vi "read_dust_control_settings.vi"(7 "Settings to be loaded":i32, 8 "error in (no error)":errorcluster, 9 "Cluster":T1, 10 "Lower Timestamp Range":timestamp, 11 "Upper Timestamp Range":timestamp) -> (0 "error out":errorcluster, 1 "Array":cluster{"String":string, "Value":dbl}[](array[cluster]), 3 "Dust Source Array":T2[](array[typedef]) {"Needle Voltage" min=0.0 max=10.0 step=0.01 format="%.2g"; "Y Voltage" min=0.0 max=9.0 step=0.01 format="%.2g"; "X Voltage" min=0.0 max=9.0 step=0.01 format="%.2g"; "Einzel Voltage" min=0.0 max=10.0 step=0.01 format="%.2g"; "Desired Amplitude (V)" min=0.0 max=10.0 step=0.01 format="%5.2f"; "Width (ms) : 0.1" min=0.05 max=5.0 step=0.01 format="%6.2f"; "Frequency" min=1.0 max=100.0 step=0.01 format="%.1f"})   [LabVIEW 2013]
uses:
  Controls/dust_soruce_control.ctl
  <vilib>/addons/database/Auxilliary.llb/DB Tools Cursor Type.ctl
  <vilib>/addons/database/Connection.llb/Conn Execute.vi
  <vilib>/addons/database/Recordset.llb/Rec Fetch Recordset Data (R).vi
  <vilib>/addons/database/Recordset.llb/Rec Destroy - Connection.vi
  <vilib>/addons/database/_DB Variant To Data/Database Variant To Data.xnode
  <vilib>/addons/database/NI_Database_API.lvlib
panel:
  out "Settings ID 2":dbl(ring) caption="Settings ID" items=["Auto", "Auto", "Auto", "Auto", "Auto", "Auto", "Auto", "Auto", "Auto", "Auto", "Auto", "Auto", "Auto", "Auto", "Auto", "Auto", "Auto", "Auto", "Auto", "Auto", "Auto test", "Auto", "Automatic Update at  10/19/2012 4:35:52 PM", "Automatic Update at  10/19/2012 4:37:24 PM", "Automatic Update at  10/19/2012 4:37:56 PM", "Automatic Update at  10/19/2012 4:39:59 PM", "Automatic Update at  10/19/2012 4:40:46 PM", "Automatic Update at  10/19/2012 4:43:56 PM", "Automatic Update at  10/19/2012 5:03:34 PM", "Awesome settings that work", "Awesome settings that work", "Automatic Update at  10/19/2012 5:32:08 PM", "Automatic Update at  10/19/2012 5:34:15 PM", "Automatic Update at  10/19/2012 5:39:51 PM", "Working settings", "Working settings", "Working settings", "Working settings", "Working settings", "Automatic Update at  10/22/2012 1:18:52 PM", "Automatic Update at  10/22/2012 1:22:32 PM", "", "Test", "Test", "Automatic Update at  10/22/2012 1:29:56 PM", "Test", "Test 1", "Test 1", "Anna's Settings", "Automatic Update at  10/22/2012 3:57:19 PM", "test of width", "Automatic Update at  10/22/2012 4:02:00 PM", "Automatic Update at  10/22/2012 4:10:30 PM", "Automatic Update at  10/22/2012 4:15:00 PM", "Automatic Update at  10/22/2012 4:38:33 PM", "Automatic Update at  10/22/2012 4:44:48 PM", "Automatic Update at  10/22/2012 4:46:11 PM", "Automatic Update at  10/22/2012 4:51:36 PM", "Automatic Update at  10/22/2012 4:54:36 PM", "Automatic Update at  10/22/2012 4:59:09 PM", "Automatic Update at  10/22/2012 5:01:02 PM", "Automatic Update at  10/22/2012 5:06:29 PM", "Automatic Update at  10/22/2012 5:13:46 PM", "Automatic Update at  10/22/2012 5:18:54 PM", "Automatic Update at  10/22/2012 5:27:58 PM", "Automatic Update at  10/22/2012 5:37:45 PM", "Automatic Update at  10/22/2012 5:39:44 PM", "Automatic Update at  10/22/2012 5:41:21 PM", "Automatic Update at  10/22/2012 5:41:55 PM", "Automatic Update at  10/22/2012 5:43:41 PM", "Automatic Update at  10/22/2012 5:45:31 PM", "Anna's Settings (Updated with working Giraffes)", "Anna's Settings (Updated with working Giraffes)", "Automatic Update at  10/23/2012 1:01:38 PM", "test", "test", "test 1", "test 1", "Automatic Update at  10/23/2012 1:44:56 PM", "Automatic Update at  10/23/2012 1:52:29 PM", "Automatic Update at  10/23/2012 1:59:24 PM", "test 3", "test 4", "Automatic Update at  10/23/2012 2:20:20 PM", "Automatic Update at  10/23/2012 5:53:49 PM", "Anna's Settings", "Anna's Settings1", "test mctesty", "test mctesty", "Automatic Update at  10/24/2012 3:47:44 PM", "Test\"", "Test\"", "this is a \"test\" setting", "Automatic Update at  10/24/2012 4:13:56 PM"]
  out "SQL Query Sintax":string
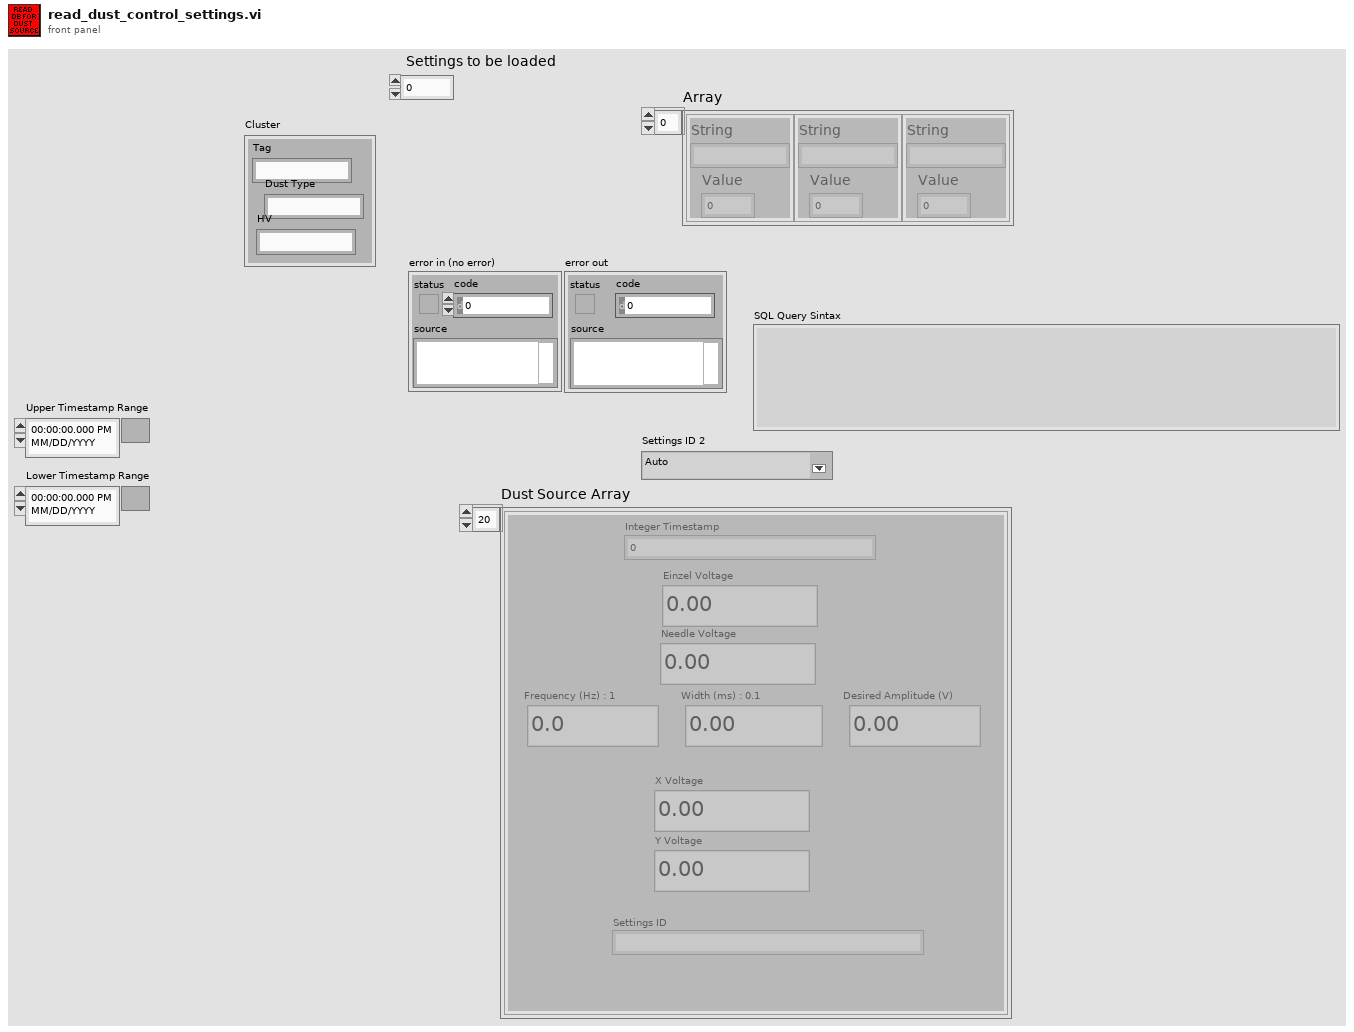
[diagram p1: front panel]
types:
  T1 = cluster{"Tag":string, "Dust Type":string, "HV":string}
  T2 = typedef "dust_soruce_control.ctl" = cluster{"Integer Timestamp":u64, "Einzel Voltage":dbl, "Needle Voltage":dbl, "Frequency":dbl, "Width (ms) : 0.1 ":dbl, "Desired Amplitude (V)":dbl, "X Voltage":dbl, "Y Voltage":dbl, "Settings ID":string, "ID#":i32}
  T3 = typedef "NI_Database_API.lvlib/DB Tools Cursor Type.ctl" = enum16{"forward-only", "keyset", "dynamic", "static"}
  T4 = typedef "NI_Database_API.lvlib/Conn ObjectReference.ctl" = refnum<k1>
  T5 = typedef "NI_Database_API.lvlib/Rec ObjectReference.ctl" = refnum<k1>
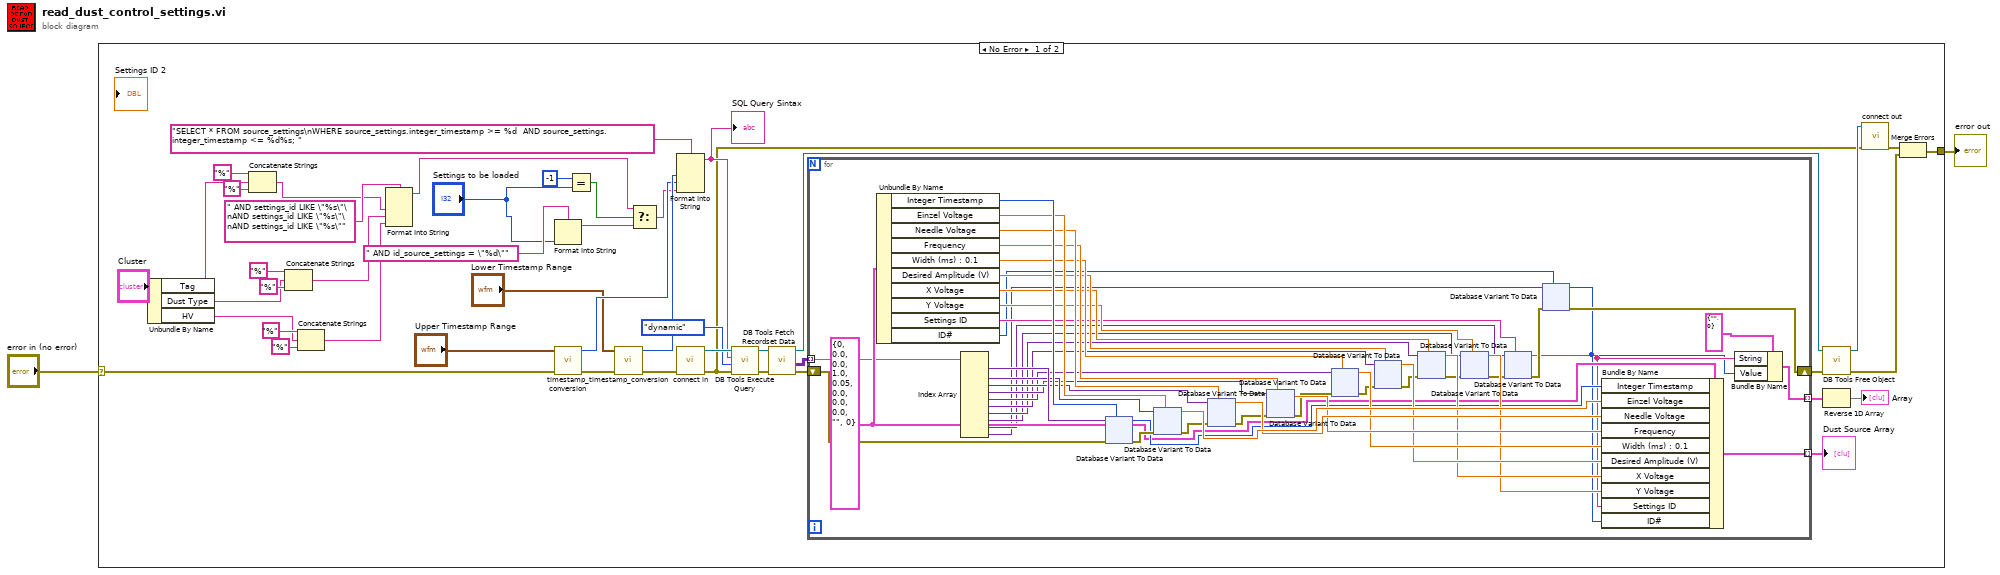
[diagram p0: block diagram]
diagram:
  n1 = case shown="No Error" "error in (no error)" {
    selector: "error in (no error)" -> [w39 w415]
    tunnel: [w22 w415] -> w1
    frame No Error {
      n2 = Unbundle By Name("Cluster") -> ("Tag"=w11:string, "Dust Type"=w6:string, "HV"=w7:string)
      n3 = Concatenate Strings("%" ("string"), w11, "%" ("string")) -> (w14:string)
      n4 = Concatenate Strings("%" ("string"), w6, "%" ("string")) -> (w4:string)
      n5 = Concatenate Strings("%" ("string"), w7, "%" ("string")) -> (w3:string)
      n6 = Format Into String(format string=" AND settings_id LIKE \"%s\"\nAND settings_id LIKE \"%s\"\nAND settings_id LIKE \"%s\"" ("string"), w14, w4, w3) -> (resulting string=w13:string)  [unwired: 2 in, 1 out]
      n7 = Format Into String(format string=" AND id_source_settings = \"%d\"" ("string"), "Settings to be loaded") -> (resulting string=w35:string)  [unwired: 2 in, 1 out]
      n8 = call "timestamp_conversion.vi"("error in (no error)"=w39, "Time Stamp"="Upper Timestamp Range") -> ("error out"=w40:errorcluster, "Integer Time"=w33:i64)  [unwired: 7 in]
      n9 = Equal?(x=-1, y="Settings to be loaded") -> (x = y?=w41:bool)
      n10 = call "timestamp_conversion.vi"("error in (no error)"=w40, "Time Stamp"="Lower Timestamp Range") -> ("error out"=w37:errorcluster, "Integer Time"=w34:i64)  [unwired: 7 in]
      n11 = Select(t=w13, s=w41, f=w35) -> (s? t:f=w27:string)
      n12 = Format Into String(format string="SELECT * FROM source_settings\nWHERE source_settings.integer_timestamp >= %d  AND source_settings.integer_timestamp <= %d%s; " ("string"), w34, w33, w27) -> (resulting string=w31:string)  [unwired: 2 in, 1 out]
      "SQL Query Sintax" <- w31
      n13 = call "connect in.vi"("error in (no error)"=w37) -> ("error out"=w20:errorcluster, "Database Connection"=w43:T4)  [unwired: 6 in, 1 out]
      n14 = call-poly <vilib>:"DB Tools Execute Query.vi"("error in (no error)"=w20, "cursor type"=DB_Tools_Cursor_Type."dynamic", "SQL query"=w31, "connection reference"=w43) -> ("error out"=w47:errorcluster, "recordset reference"=w48:T5)  [unwired: 4 in]
      n15 = call-poly <vilib>:"DB Tools Fetch Recordset Data.vi"("error in (no error)"=w47, "recordset reference"=w48) -> ("error out"=w45:errorcluster, "recordset data"=w38:variant[][], "recordset reference out"=w46:T5)  [unwired: 3 in]
      n16 = for {
        tunnel: w38 -> [w75] mode=indexing
        shift-right: [w55] -> w44
        shift-left: w45 -> [w94]
        tunnel: [w78] -> w26 mode=indexing
        tunnel: [w51] -> w25 mode=indexing
        w76 = T2 {"Integer Timestamp"=0, "Einzel Voltage"=0.0, "Needle Voltage"=0.0, "Frequency"=1.0, "Width (ms) : 0.1 "=0.05, "Desired Amplitude (V)"=0.0, "X Voltage"=0.0, "Y Voltage"=0.0, "Settings ID"="", "ID#"=0} ("Dust Source Controls")
        n17 = Unbundle By Name(w76) -> ("Integer Timestamp"=w74:u64, "Einzel Voltage"=w72:dbl, "Needle Voltage"=w70:dbl, "Frequency"=w68:dbl, "Width (ms) : 0.1"=w66:dbl, "Desired Amplitude (V)"=w63:dbl, "X Voltage"=w61:dbl, "Y Voltage"=w60:dbl, "Settings ID"=w58:string, "ID#"=w53:i32)
        n18 = Index Array(array=w75) -> (element #1=w73:variant, element #2=w71:variant, element #3=w69:variant, element #4=w67:variant, element #5=w65:variant, element #6=w64:variant, element #7=w62:variant, element #8=w59:variant, element #9=w57:variant, element #10=w54:variant)  [unwired: 10 in]
        n19 = xnode "Database Variant To Data"("database variant"=w73, "error in"=w94, "type"=w74) -> ("data"=w77:u64, "error out"=w92:errorcluster)
        n20 = xnode "Database Variant To Data"("database variant"=w71, "error in"=w92, "type"=w72) -> ("data"=w93:dbl, "error out"=w90:errorcluster)
        n21 = xnode "Database Variant To Data"("database variant"=w69, "error in"=w90, "type"=w70) -> ("data"=w91:dbl, "error out"=w88:errorcluster)
        n22 = xnode "Database Variant To Data"("database variant"=w67, "error in"=w88, "type"=w68) -> ("data"=w89:dbl, "error out"=w86:errorcluster)
        n23 = xnode "Database Variant To Data"("database variant"=w65, "error in"=w86, "type"=w66) -> ("data"=w87:dbl, "error out"=w85:errorcluster)
        n24 = xnode "Database Variant To Data"("database variant"=w64, "error in"=w85, "type"=w63) -> ("data"=w84:dbl, "error out"=w82:errorcluster)
        n25 = xnode "Database Variant To Data"("database variant"=w62, "error in"=w82, "type"=w61) -> ("data"=w83:dbl, "error out"=w80:errorcluster)
        n26 = xnode "Database Variant To Data"("database variant"=w59, "error in"=w80, "type"=w60) -> ("data"=w81:dbl, "error out"=w79:errorcluster)
        n27 = xnode "Database Variant To Data"("database variant"=w57, "error in"=w79, "type"=w58) -> ("data"=w50:string, "error out"=w56:errorcluster)
        n28 = xnode "Database Variant To Data"("database variant"=w54, "error in (no error)"=w56, "type"=w53) -> ("data"=w49:i32, "error out"=w55:errorcluster)
        n29 = Bundle By Name(cluster=w76, "Integer Timestamp"=w77, "Einzel Voltage"=w93, "Needle Voltage"=w91, "Frequency"=w89, "Width (ms) : 0.1"=w87, "Desired Amplitude (V)"=w84, "X Voltage"=w83, "Y Voltage"=w81, "Settings ID"=w50, "ID#"=w49) -> (w78:T2)
        n30 = Bundle By Name(cluster=cluster{"String":string, "Value":i32} {"String"="", "Value"=0}, "String"=w50, "Value"=w49) -> (w51:cluster{"String":string, "Value":i32})
      }
      "Dust Source Array" <- w26
      n31 = call-poly <vilib>:"DB Tools Free Object.vi"("error in (no error)"=w44, "recordset reference"=w46) -> ("error out"=w21:errorcluster, "connection reference"=w42:T4)  [unwired: 8 in]
      n32 = Reverse 1D Array(array=w25) -> (reversed array=→"Array":cluster{"String":string, "Value":i32}[])
      n33 = call "connect out.vi"("error in (no error)"=w20, "connection reference"=w42) -> ("error out"=w23:errorcluster)  [unwired: 9 in]
      n34 = Merge Errors(w23, w21) -> (w22:errorcluster)
    }
    frame Error {
    }
  }
  "error out" <- w1
